vi "Message.vi"(8 "error in (no error)":errorcluster, 9 "Message":T1, 10 "Service":T2, 11 "MicronCLI in":refnum<class "MicronCLI.lvclass">) -> (0 "error out":errorcluster, 2 "Response":string, 3 "MicronCLI out":refnum<class "MicronCLI.lvclass">)   [LabVIEW 2019, in "MicronCLI.lvclass"]
uses:
  MicronCLI.lvclass
  Typedefs/ServiceDetails.ctl
  Typedefs/Message.ctl
  MicronCLI.lvclass/MicronCLI.ctl
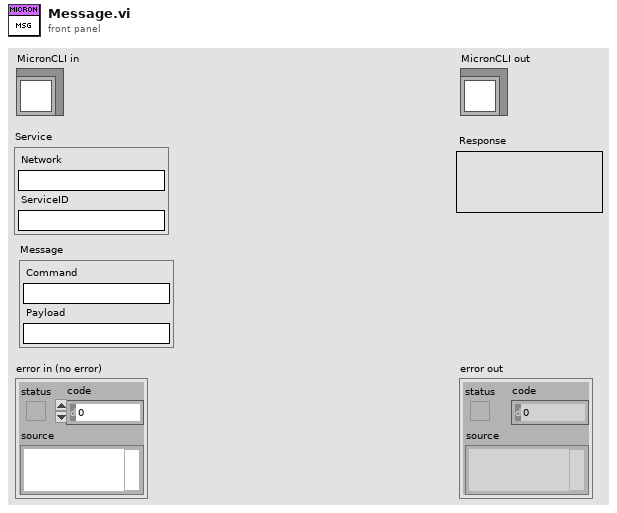
[diagram p1: front panel]
types:
  T1 = typedef "MicronCLI.lvclass/Message.ctl" = cluster{"Command":string, "Payload":string}
  T2 = typedef "MicronCLI.lvclass/ServiceDetails.ctl" = cluster{"Network":string, "ServiceID":string}
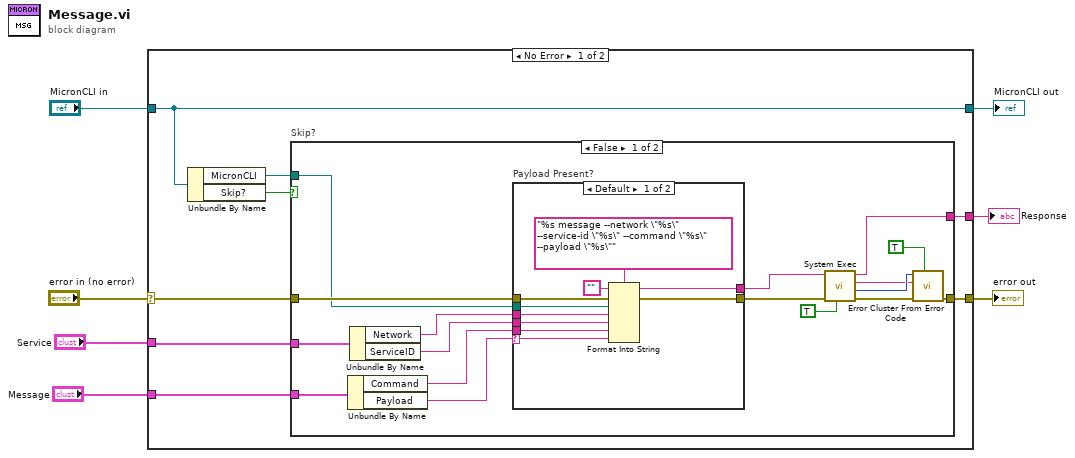
[diagram p0: block diagram]
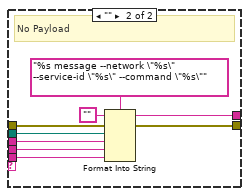
[diagram p2: hidden frame]
diagram:
  n1 = case shown="No Error" "error in (no error)" {
    selector: "error in (no error)" -> [w15 w54]
    tunnel: [w11 w54] -> w6
    tunnel: [w14 w53] -> w4
    tunnel: "MicronCLI in" -> [w14 w53]
    tunnel: "Service" -> [w12 _]
    tunnel: "Message" -> [w9 _]
    tunnel: [w8 _] -> w1
    frame No Error {
      n2 = Unbundle By Name(w14) -> ("MicronCLI"=w13:path, "Skip?"=w10:bool)
      n3 = case "Skip?" shown="False" w10 {
        tunnel: w15 -> [w32 w52]
        tunnel: w13 -> [w29 _]
        tunnel: w12 -> [w28 _]
        tunnel: [w23 w52] -> w11
        tunnel: w9 -> [w19 _]
        tunnel: [w16 _] -> w8
        frame False {
          n4 = Unbundle By Name(w19) -> ("Command"=w18:string, "Payload"=w17:string)
          n5 = Unbundle By Name(w28) -> ("Network"=w27:string, "ServiceID"=w26:string)
          n6 = case "Payload Present?" shown="Default" w17 {
            selector: w17 -> [w33 _]
            tunnel: w32 -> [w42 w51]
            tunnel: [w41 w50] -> w30
            tunnel: w29 -> [w39 w48]
            tunnel: w27 -> [w37 w46]
            tunnel: w26 -> [w36 w45]
            tunnel: [w35 w44] -> w25
            tunnel: w18 -> [w34 w43]
            frame Default {
              n7 = Format Into String(format string="%s message --network \"%s\" --service-id \"%s\" --command \"%s\" --payload \"%s\"", initial string="", error in=w42, w39, w37, w36, w34, w33) -> (resulting string=w35:string, error out=w41:errorcluster)
            }
            frame "" {
              # "No Payload"
              n8 = Format Into String(format string="%s message --network \"%s\" --service-id \"%s\" --command \"%s\"", initial string="", error in=w51, w48, w46, w45, w43) -> (resulting string=w44:string, error out=w50:errorcluster)
            }
          }
          n9 = call <vilib>:"System Exec.vi"("run minimized? (F)"=TRUE, "error in (no error)"=w30, "command line"=w25) -> ("error out"=w31:errorcluster, "return code"=w22:i32, "standard error"=w21:string, "standard output"=w16:string)  [unwired: 5 in]
          n10 = call <vilib>:"Error Cluster From Error Code.vi"("show call chain? (False)"=TRUE, "error in (no error)"=w31, "error message (\"\")"=w21, "error code (0)"=w22) -> ("error out"=w23:errorcluster)  [unwired: 5 in]
        }
        frame True {
        }
      }
    }
    frame Error {
    }
  }
  "error out" <- w6
  "MicronCLI out" <- w4
  "Response" <- w1
